vi "Get Data Name.vi"(8 "错误输入":errorcluster, 11 "Data":variant) -> (0 "错误输出":errorcluster, 2 "Data Name":string, 3 "Data dup":variant)   [LabVIEW 2012, in "TD Tools.lvlib"]
uses:
  TD Tools.lvlib
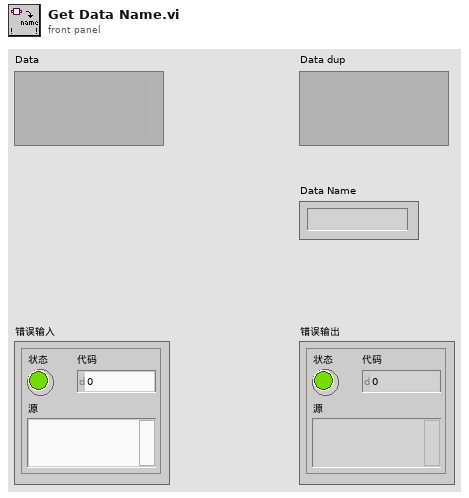
[diagram p1: front panel]
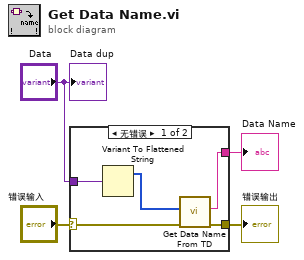
[diagram p0: block diagram]
diagram:
  n1 = case shown="无错误" "错误输入" {
    selector: "错误输入" -> [w9 w10]
    tunnel: [w8 w10] -> w3
    tunnel: "Data" -> [w7 _]
    tunnel: [w5 _] -> w1
    frame No Error {
      n2 = Variant To Flattened String(Variant=w7) -> (1:w6:i16[])  [unwired: 1 out]
      n3 = call "Get Data Name From TD.vi"("错误输入"=w9, "Type Descriptor"=w6) -> ("错误输出"=w8:errorcluster, "Name"=w5:string)  [unwired: 8 in]
    }
    frame Error {
    }
  }
  "Data Name" <- w1
  "错误输出" <- w3
  "Data dup" <- "Data"
